vi "DHE_ParserType.vi"(8 "error in (no error)":errorcluster, 9 "arguments":string, 10 "function":string, 11 "fd in":i32) -> (0 "error out":errorcluster, 1 "result type":string, 2 "str result":string, 3 "fd out":i32)   [LabVIEW 2016]
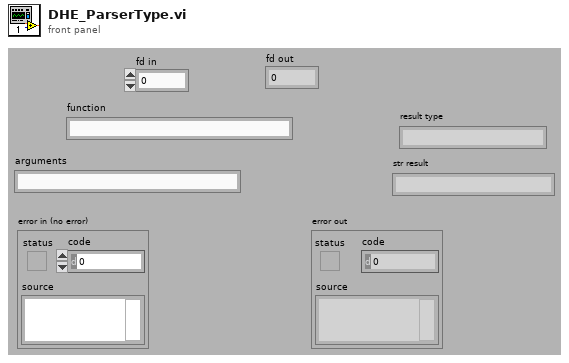
[diagram p1: front panel]
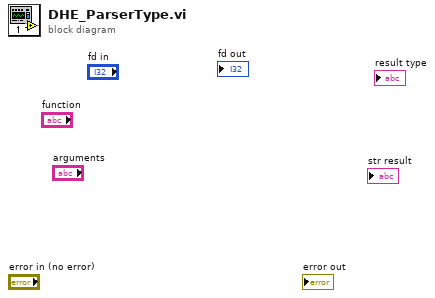
[diagram p0: block diagram]
diagram:
